vi "Enable&Disable_Controls.vi"(1 "Enum":enum16{"Enabled", "Disabled", "Disabled&Grayed"}(ring), 2 "References":refnum<vi>[](array[refnum])=[refnum, refnum, refnum, refnum, refnum, refnum, refnum, refnum, refnum, refnum]) -> ()   [LabVIEW 2019]
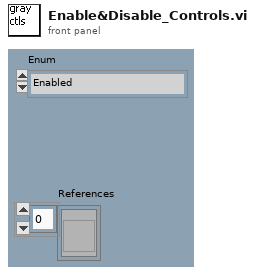
[diagram p1: front panel]
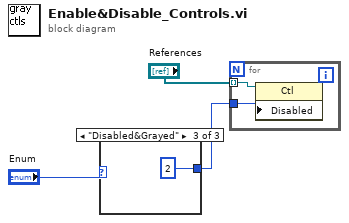
[diagram p0: block diagram]
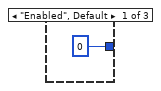
[diagram p2: hidden frame]
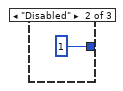
[diagram p3: hidden frame]
diagram:
  n1 = case shown="\"Disabled&Grayed\"" "Enum" {
    tunnel: [u8 0 ("Disabled") u8 1 ("Disabled") u8 2 ("Disabled")] -> w1
    frame "Enabled", Default {
    }
    frame "Disabled" {
    }
    frame "Disabled&Grayed" {
    }
  }
  n2 = for {
    tunnel: "References" -> [w8] mode=indexing
    tunnel: w1 -> [w7]
    n3 = property class="Ctl"(reference=w8, "Disabled"=w7) -> ()  [unwired: 1 in, 2 out]
  }
